vi "Ball Align(SubVI).vi"(0 "align (t-x/f-y)":refnum<vi>, 1 "defY":dbl, 2 "defX":dbl, 3 "Range":dbl, 5 "x is in range":refnum<vi>, 7 "y is in range":refnum<vi>, 11 "curX":dbl, 12 "curY":dbl, 13 "Align X - t, Y - f":bool) -> (4 "Boolean":bool, 6 "Boolean 4":bool, 8 "Boolean 3":bool, 10 "Boolean 2":bool, 14 "x_is_in_range":bool, 15 "y_is_in_range":bool)   [LabVIEW 2017]
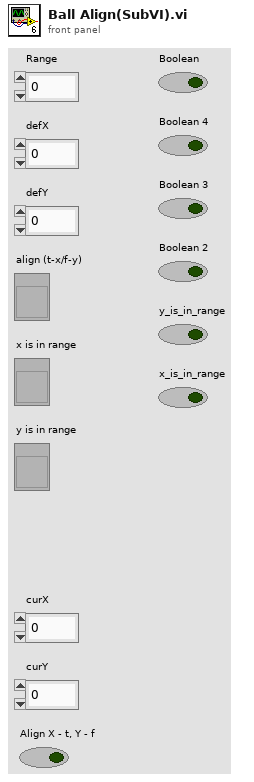
[diagram p1: front panel]
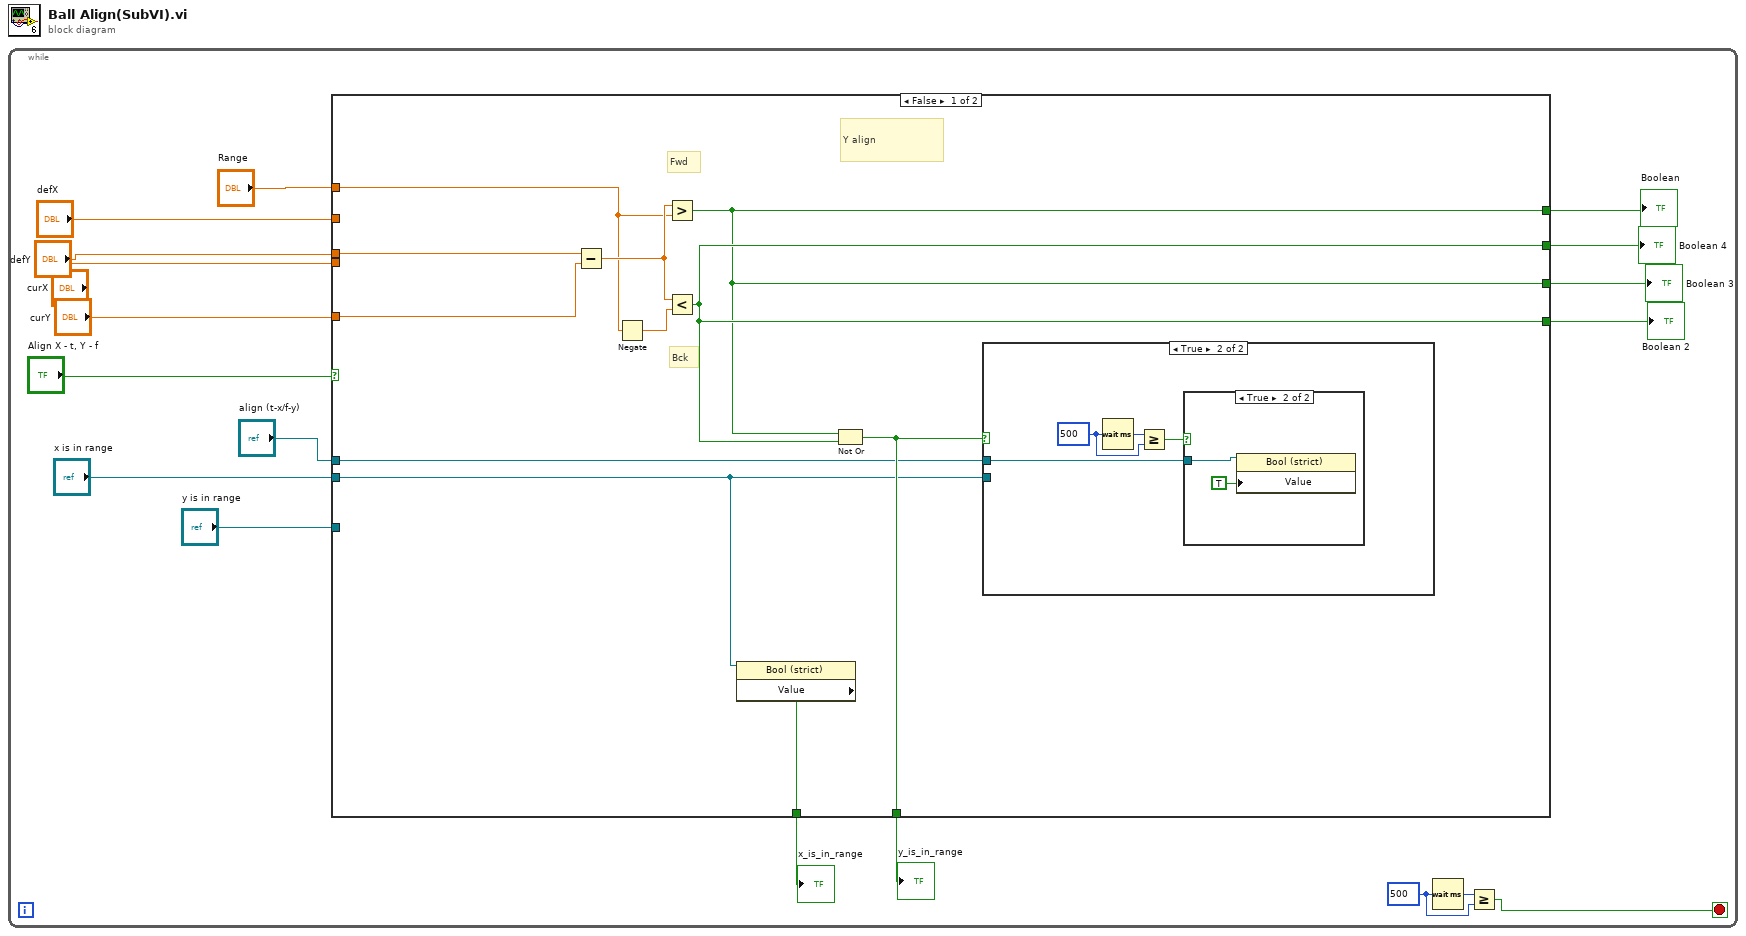
[diagram p0: block diagram]
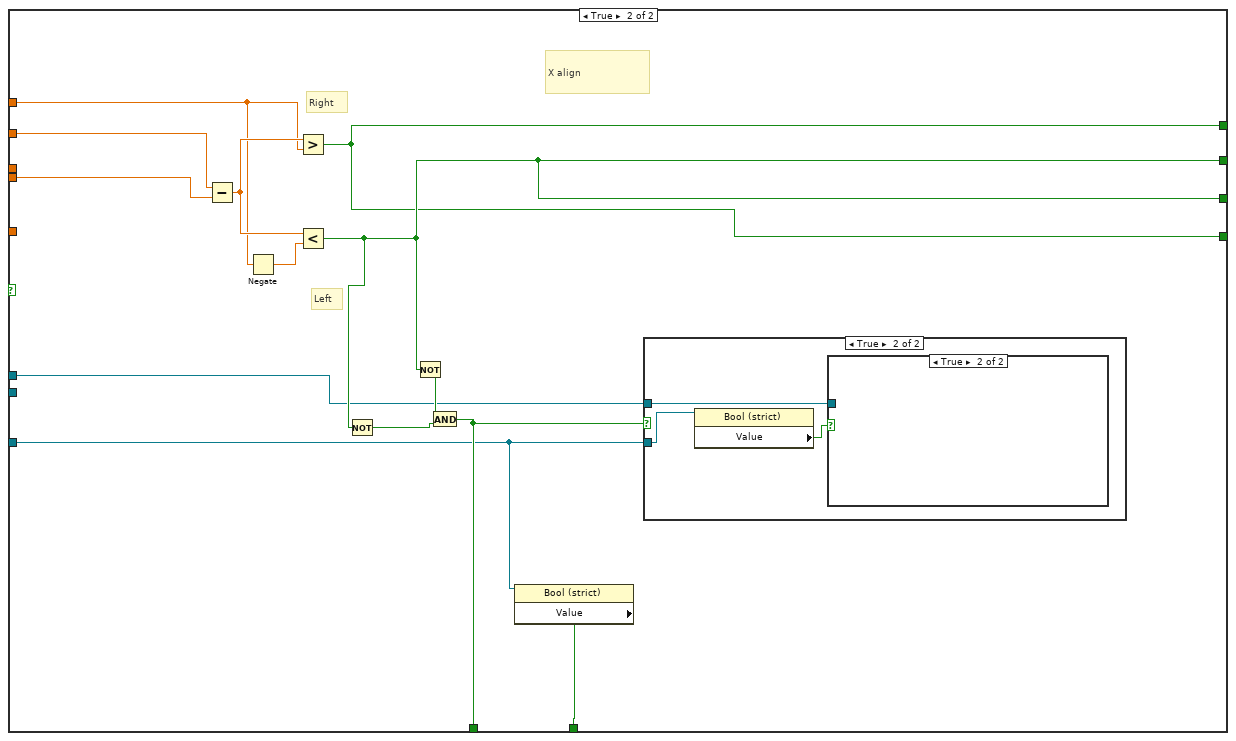
[diagram p4: hidden frame]
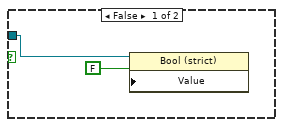
[diagram p6: hidden frame]
diagram:
  n1 = while {
    stop <- w1 stop-if-true
    w2 = u32 500 ("milliseconds to wait")
    n2 = case shown="False" "Align X - t, Y - f" {
      tunnel: "defX" -> [_ w44]
      tunnel: "curX" -> [_ w43]
      tunnel: "Range" -> [w25 w42]
      tunnel: "defY" -> [w27 _]
      tunnel: "curY" -> [w26 _]
      tunnel: [w24 w37] -> w13
      tunnel: [w20 w41] -> w14
      tunnel: [w23 w40] -> w15
      tunnel: [w22 w40] -> w16
      tunnel: [w23 w39] -> w17
      tunnel: [w22 w39] -> w18
      tunnel: "x is in range" -> [w19 _]
      tunnel: "align (t-x/f-y)" -> [w21 w38]
      tunnel: "y is in range" -> [_ w36]
      frame False {
        # "Bck"
        # "Fwd"
        # "Y align"
        n3 = Subtract(x=w27, y=w26) -> (x-y=w29:dbl)
        n4 = Negate(x=w25) -> (-x=w28:dbl)
        n5 = Greater?(x=w29, y=w25) -> (0:w22:bool)
        n6 = Less?(x=w29, y=w28) -> (x < y?=w23:bool)
        n7 = property class="Bool (strict)"(reference=w19) -> ("Value"=w20:bool)  [unwired: 1 in, 2 out]
        n8 = Not Or(1:w23, 2:w22) -> (0:w24:bool)
        n9 = case shown="True" w24 {
          tunnel: w21 -> [_ w30]
          tunnel: w19 -> [_ _]
          frame False {
          }
          frame True {
            w31 = u32 500 ("milliseconds to wait")
            n10 = Wait (ms)(milliseconds to wait=w31) -> (millisecond timer value=w32:u32)
            n11 = Greater Or Equal?(x=w32, y=w31) -> (x >= y?=w33:bool)
            n12 = case shown="True" w33 {
              tunnel: w30 -> [_ w34]
              frame False {
              }
              frame True {
                n13 = property class="Bool (strict)"(reference=w34, "Value"=TRUE ("X - t, Y - f")) -> ()  [unwired: 1 in, 2 out]
              }
            }
          }
        }
      }
      frame True {
        # "X align"
        # "Right"
        # "Left"
        n14 = Subtract(x=w44, y=w43) -> (x-y=w48:dbl)
        n15 = Negate(x=w42) -> (-x=w47:dbl)
        n16 = Greater?(x=w48, y=w42) -> (0:w39:bool)
        n17 = Less?(x=w48, y=w47) -> (x < y?=w40:bool)
        n18 = Not(x=w40) -> (.not. x?=w45:bool)
        n19 = Not(x=w40) -> (.not. x?=w46:bool)
        n20 = And(x=w46, y=w45) -> (x .and. y?=w41:bool)
        n21 = property class="Bool (strict)"(reference=w36) -> ("Value"=w37:bool)  [unwired: 1 in, 2 out]
        n22 = case shown="True" w41 {
          tunnel: w38 -> [_ w50]
          tunnel: w36 -> [_ w49]
          frame False {
          }
          frame True {
            n23 = property class="Bool (strict)"(reference=w49) -> ("Value"=w51:bool)  [unwired: 1 in, 2 out]
            n24 = case shown="True" w51 {
              tunnel: w50 -> [w52 _]
              frame False {
                n25 = property class="Bool (strict)"(reference=w52, "Value"=FALSE ("X - t, Y - f")) -> ()  [unwired: 1 in, 2 out]
              }
              frame True {
              }
            }
          }
        }
      }
    }
    "Boolean" <- w18
    "Boolean 2" <- w17
    "Boolean 3" <- w16
    "Boolean 4" <- w15
    "x_is_in_range" <- w14
    "y_is_in_range" <- w13
    n26 = Wait (ms)(milliseconds to wait=w2) -> (millisecond timer value=w3:u32)
    n27 = Greater Or Equal?(x=w3, y=w2) -> (x >= y?=w1:bool)
  }
